vi "Stop All.vi"(8 "error in (no error)":errorcluster, 11 "Motions in":refnum<class "Motions.lvclass">) -> (0 "error out":errorcluster, 3 "Motions out":refnum<class "Motions.lvclass">)   [LabVIEW 2016, in "Hardware.lvlib" / "Motions.lvlib" / "Motions.lvclass"]
uses:
  <userlib>/Common Components/Hardware/Abstract System/Motions/Motions/Motions.lvclass
  <userlib>/Common Components/Hardware/Abstract System/Motions/Motions/Motions.lvclass/Motions.ctl
  <userlib>/Common Components/Hardware/Motor/Motor/Motor.lvclass
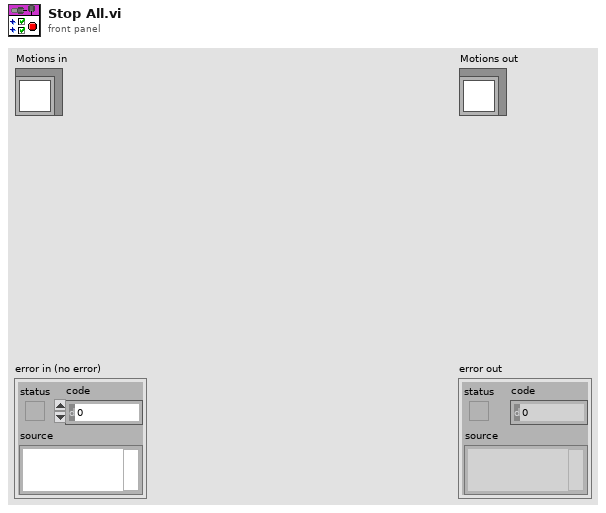
[diagram p1: front panel]
types:
  T1 = typedef "Hardware.lvlib/Motions.lvlib/Motions.lvclass/Motor States.ctl" = cluster{"Connected":bool, "Enabled":bool, "Moving Status":bool, "Soft Moving Status":bool, "Current Pos":dbl, "Target Pos":dbl, "Moving Dir (-1, 0, 1)":i32, "Error Status":bool, "Hard Limit+":bool, "Hard Limit-":bool, "Soft Limit+":bool, "Soft Limit-":bool, "Motion Dst Queue":refnum<queue>, "History Dst Stack":refnum<queue>}
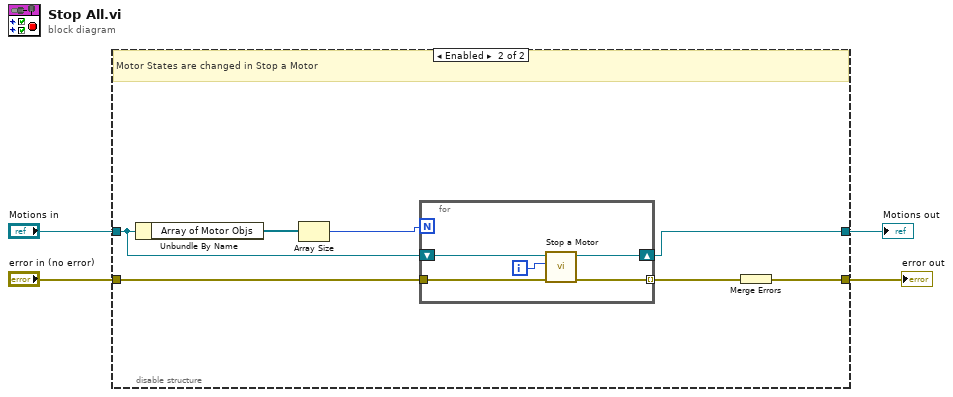
[diagram p0: block diagram]
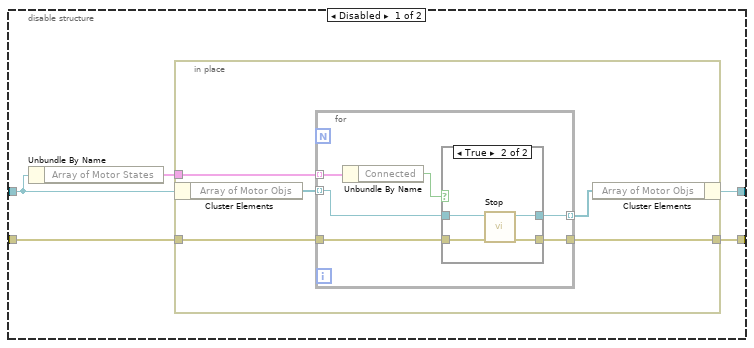
[diagram p2: hidden frame]
diagram:
  n1 = disable-structure shown="Enabled" {
    disable-tunnel: [w9 w32] -> w4
    disable-tunnel: "error in (no error)" -> [w8 w29]
    disable-tunnel: [w7 w27] -> w2
    disable-tunnel: "Motions in" -> [w6 w33]
    frame Disabled {
      n2 = Unbundle By Name(w6) -> ("Array of Motor States"=w5:T1[])
      n3 = in-place {
        in-place-border: w8 -> [w14]
        in-place-border: [w13] -> w7
        in-place-border: w5 -> [w10]
        n4 = in-place-cluster #1(w6) -> ("Array of Motor Objs"=w12:refnum<class "Motor.lvclass">[])
        n5 = for {
          tunnel: w14 -> [w20]
          tunnel: [w19] -> w13
          tunnel: w12 -> [w18] mode=indexing
          tunnel: [w17] -> w11 mode=indexing
          tunnel: w10 -> [w16] mode=indexing
          n6 = Unbundle By Name(w16) -> ("Connected"=w15:bool)
          n7 = case shown="True" w15 {
            tunnel: w20 -> [w21 w26]
            tunnel: [w21 w25] -> w19
            tunnel: w18 -> [w22 w24]
            tunnel: [w22 w23] -> w17
            frame False {
            }
            frame True {
              n8 = call-dynamic "Stop.vi"("error in (no error)"=w26, "Motor in"=w24) -> ("error out"=w25:errorcluster, "Motor out"=w23:refnum<class "Motor.lvclass">)  [unwired: 8 in]
            }
          }
        }
        n9 = in-place-cluster #1("Array of Motor Objs"=w11) -> (w9:refnum<class "Motions.lvclass">)
      }
    }
    frame Enabled {
      # "Motor States are changed in Stop a Motor"
      n10 = Unbundle By Name(w33) -> ("Array of Motor Objs"=w31:refnum<class "Motor.lvclass">[])
      n11 = Array Size(array=w31) -> (size(s)=w30:i32)
      n12 = for {
        N: w30 -> [_]
        shift-right: [w37] -> w32
        shift-left: w33 -> [w38]
        tunnel: w29 -> [w35]
        tunnel: [w34] -> w28 mode=indexing
        i -> [w36]
        n13 = call <userlib>:"Stop a Motor.vi"("error in (no error)"=w35, "index"=w36, "Motions in"=w38) -> ("error out"=w34:errorcluster, "Motions out"=w37:refnum<class "Motions.lvclass">)  [unwired: 7 in]
      }
      n14 = Merge Errors(w28) -> (w27:errorcluster)
    }
  }
  "error out" <- w2
  "Motions out" <- w4
